vi "Filtered_read_of_file.vi"(4 "Data string":string, 5 "End Of File already Reached?":bool, 6 "Start of data (bytes)":i32, 7 "Desired Channel names":string[](array[string]), 8 "Valid Channel Options":string[][](array[string]), 9 "All Channels Present":string[](array[string]), 10 "Filename":path) -> (2 "Output Values":string[][](array[string]))   [LabVIEW 2010]
uses:
  Data_plotting_vis/Results_plotter_Global.vi
panel:
  out "Case":string
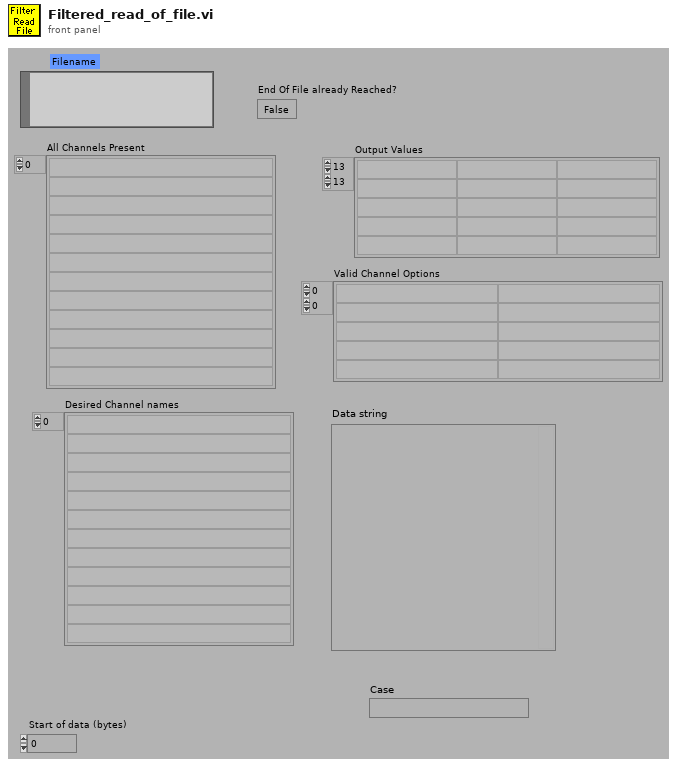
[diagram p1: front panel]
types:
  T1 = enum16{"read/write", "read-only", "write-only", "write-only (truncate)"}
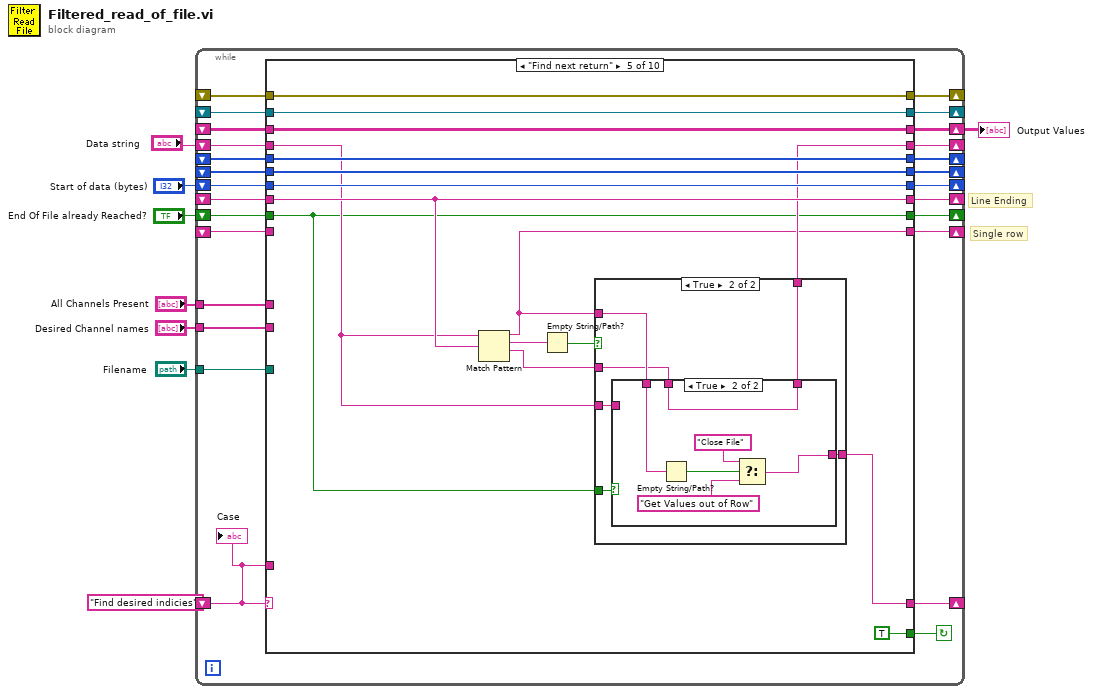
[diagram p0: block diagram]
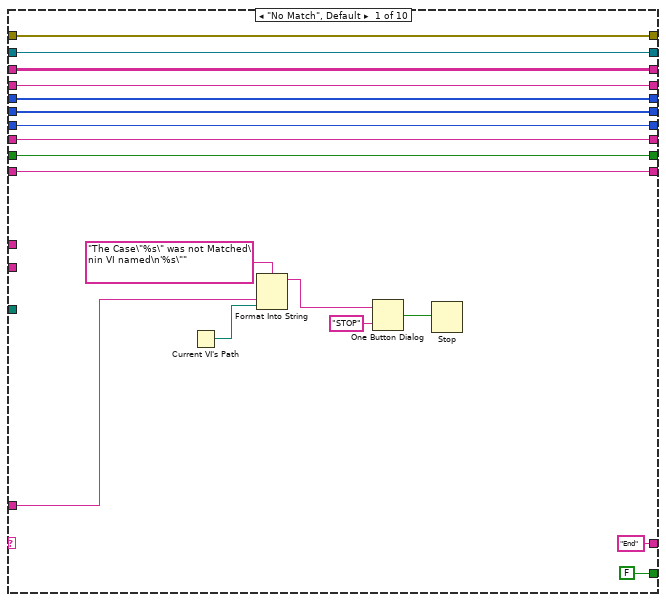
[diagram p2: hidden frame]
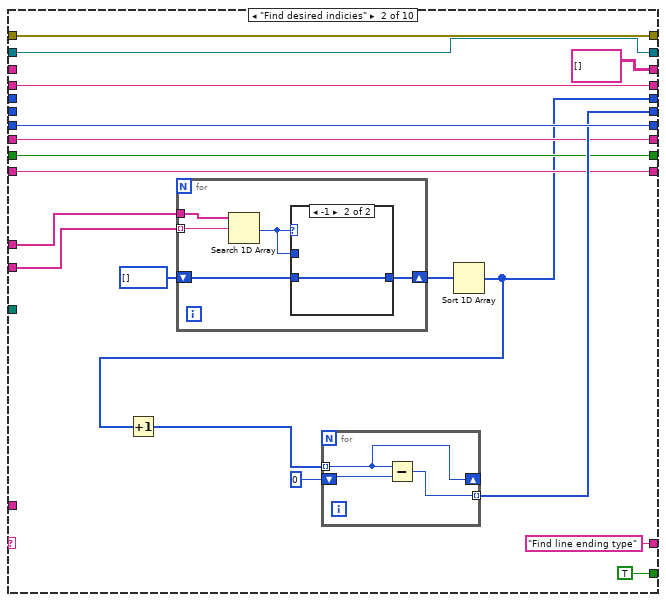
[diagram p3: hidden frame]
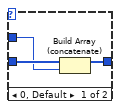
[diagram p4: hidden frame]
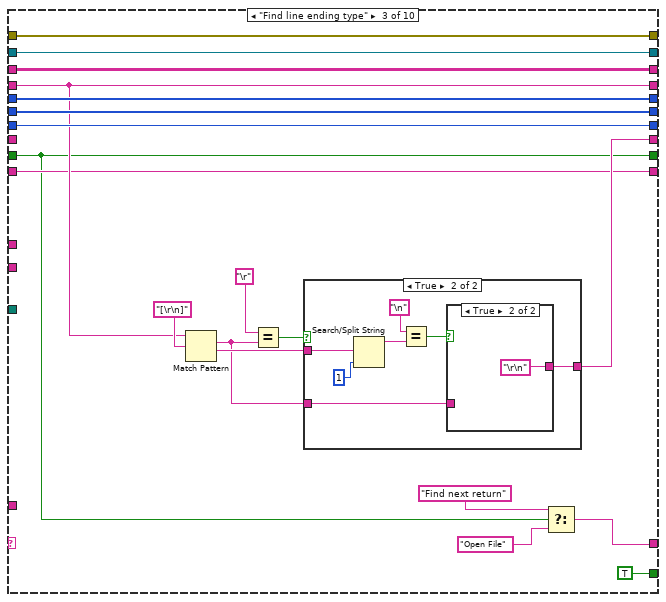
[diagram p5: hidden frame]
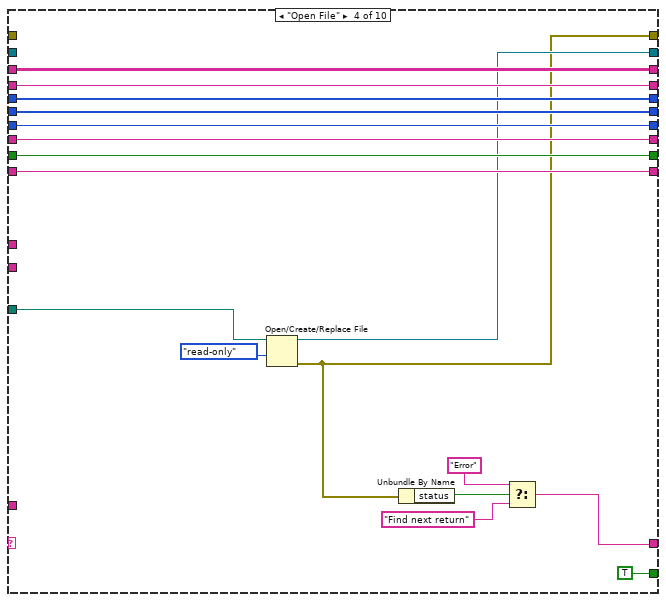
[diagram p8: hidden frame]
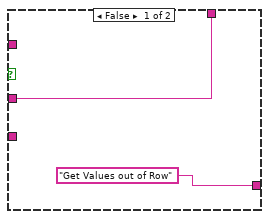
[diagram p9: hidden frame]
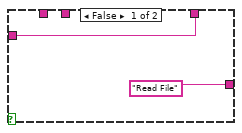
[diagram p10: hidden frame]
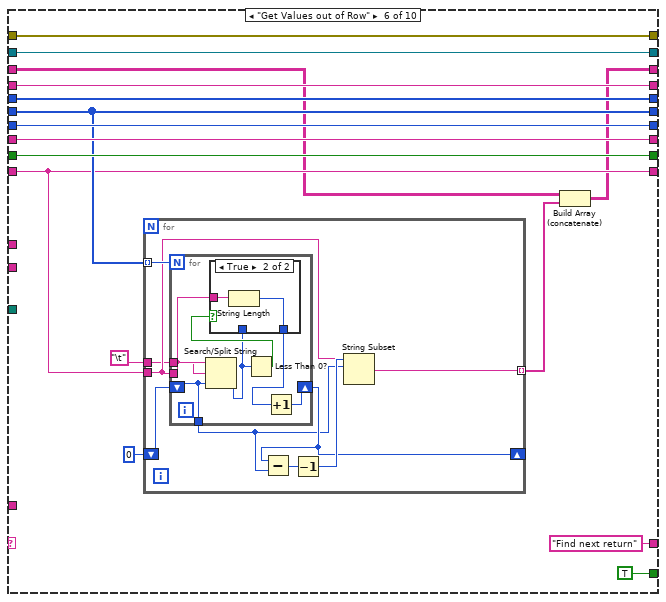
[diagram p11: hidden frame]
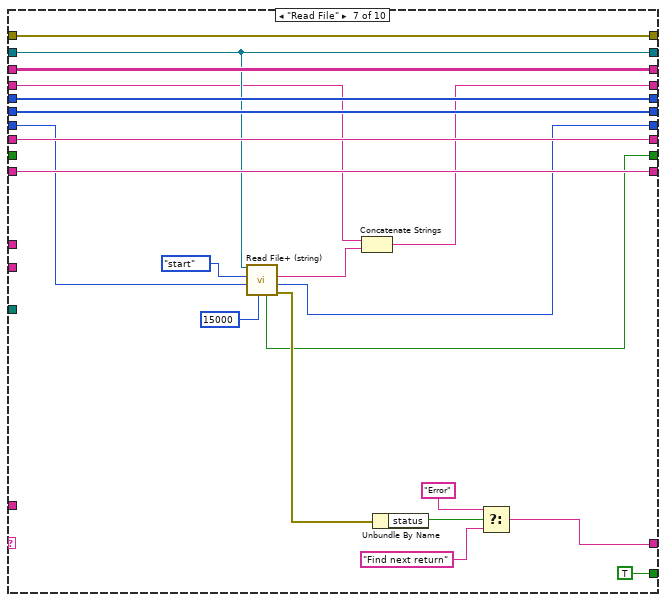
[diagram p13: hidden frame]
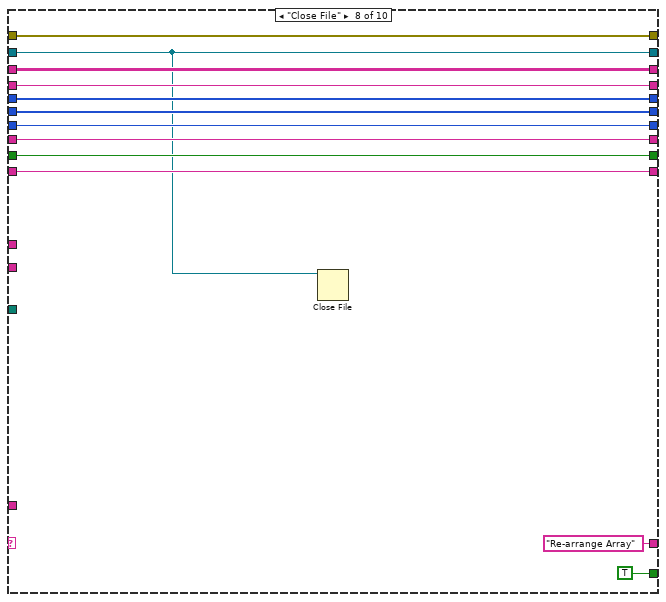
[diagram p14: hidden frame]
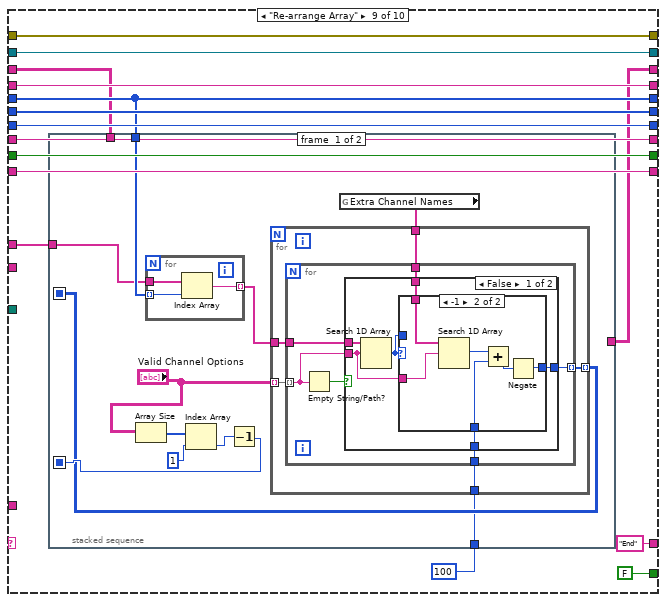
[diagram p15: hidden frame]
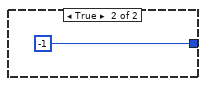
[diagram p17: hidden frame]
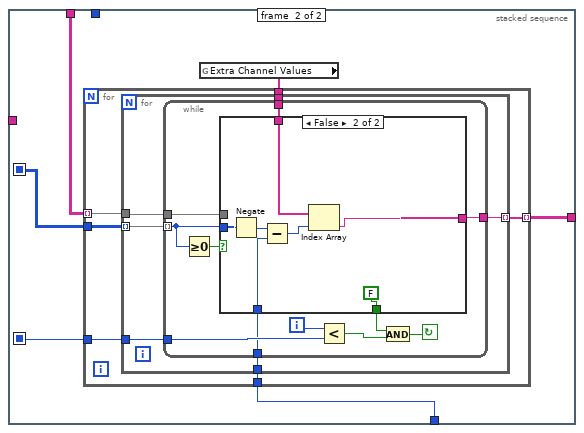
[diagram p18: hidden frame]
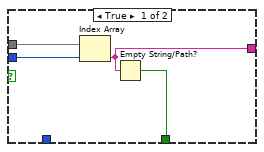
[diagram p19: hidden frame]
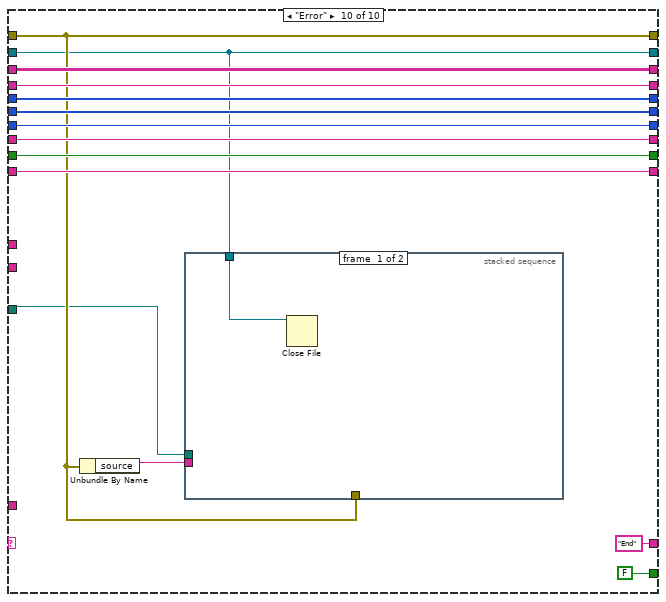
[diagram p20: hidden frame]
diagram:
  # "Single row"
  # "Line Ending"
  n1 = while {
    tunnel: "Filename" -> [w10]
    shift-left: _ -> [w12]
    shift-right: [w11] -> _
    shift-left: _ -> [w14]
    shift-right: [w13] -> _
    shift-left: _ -> [w16]
    shift-right: [w15] -> w2
    shift-left: "End Of File already Reached?" -> [w18]
    shift-right: [w17] -> _
    shift-left: _ -> [w19]
    shift-right: [w20] -> _
    shift-left: _ -> [w21]
    shift-right: [w22] -> _
    tunnel: "All Channels Present" -> [w23]
    tunnel: "Desired Channel names" -> [w9]
    shift-left: "Data string" -> [w25]
    shift-right: [w24] -> _
    shift-left: _ -> [w27]
    shift-right: [w26] -> _
    shift-left: "Start of data (bytes)" -> [w29]
    shift-right: [w28] -> _
    shift-left: _ -> [w30]
    shift-right: [w31] -> _
    shift-left: "Find desired indicies" -> [w33]
    shift-right: [w32] -> _
    stop <- w34 continue-if-true
    n2 = case shown="\"Find next return\"" w33 {
      tunnel: [FALSE ("Results File?") TRUE ("Results File?") TRUE ("Results File?") TRUE ("Results File?") TRUE ("Results File?") TRUE ("Results File?") TRUE ("Results File?") TRUE ("Results File?") FALSE ("Results File?") FALSE ("Results File?")] -> w34
      tunnel: w33 -> [w47 _ _ _ _ _ _ _ _ _]
      tunnel: ["End" "Find line ending type" ("f") w83 w113 w132 "Find next return" ("f") w200 "Re-arrange Array" ("f") "End" ("f") "End" ("f")] -> w32
      tunnel: [w44 w61 w100 w126 w143 w169 w215 w226 w242 w334] -> w31
      tunnel: w30 -> [w44 _ w100 w126 w143 w169 w215 w226 w242 w334]
      tunnel: w29 -> [w43 w68 w99 w125 w142 w174 w206 w225 w241 w333]
      tunnel: [w43 w68 w99 w125 w142 w174 w205 w225 w241 w333] -> w28
      tunnel: w27 -> [w42 _ w101 w127 w144 w175 w216 w227 w233 w335]
      tunnel: [w42 w54 w101 w127 w144 w175 w216 w227 w233 w335] -> w26
      tunnel: w25 -> [w41 w67 w93 w128 w136 w176 w198 w228 w243 w336]
      tunnel: [w41 w67 w93 w128 w137 w176 w196 w228 w243 w336] -> w24
      tunnel: w9 -> [_ w64 _ _ _ _ _ _ _ _]
      tunnel: w23 -> [_ w63 _ _ _ _ _ _ w232 _]
      tunnel: [w40 w60 w91 w123 w140 w171 w213 w223 w239 w330] -> w22
      tunnel: w21 -> [w40 w60 _ w123 w140 w171 w213 w223 w239 w330]
      tunnel: [w39 w59 w90 w122 w129 w168 w212 w222 w238 w329] -> w20
      tunnel: w19 -> [w39 w59 w90 w122 _ w168 w212 w222 w238 w329]
      tunnel: w18 -> [w38 w58 w84 w121 w131 w170 _ w221 w237 w328]
      tunnel: [w38 w58 w84 w121 w131 w170 w199 w221 w237 w328] -> w17
      tunnel: w16 -> [w37 _ w89 w120 w135 w164 w211 w220 w231 w327]
      tunnel: [w37 string[][] [] w89 w120 w135 w163 w211 w220 w230 w327] -> w15
      tunnel: w14 -> [w36 w56 w88 _ w134 w162 w207 w218 w235 w323]
      tunnel: [w36 w56 w88 w118 w134 w162 w207 w218 w235 w323] -> w13
      tunnel: w12 -> [w35 w55 w87 _ w133 w161 w208 w219 w236 w326]
      tunnel: [w35 w55 w87 w117 w133 w161 w208 w219 w236 w326] -> w11
      tunnel: w10 -> [_ _ _ w112 _ _ _ _ _ w324]
      frame "No Match", Default {
        n3 = Current VI's Path() -> (path=w48:path)
        n4 = Format Into String(format string="The Case\"%s\" was not Matched\nin VI named\n'%s\"" ("Format String"), w47, w48) -> (resulting string=w51:string)  [unwired: 2 in, 1 out]
        n5 = One Button Dialog(message=w51, button name ("OK")="STOP") -> (true=w49:bool)
        n6 = Stop(stop? (T)=w49) -> ()
      }
      frame "Find desired indicies" {
        n7 = for {
          tunnel: w63 -> [w78]
          tunnel: w64 -> [w77] mode=indexing
          shift-right: [w75] -> w66
          shift-left: i32[] [] -> [w76]
          n8 = Search 1D Array(1D array=w78, element=w77) -> (index of element=w74:i32)  [unwired: 1 in]
          n9 = case shown="-1" w74 {
            tunnel: w76 -> [w81 w82]
            tunnel: [w79 w82] -> w75
            tunnel: w74 -> [w80 _]
            frame 0, Default {
              n10 = Build Array (concatenate)(w81, w80) -> (w79:i32[])
            }
            frame -1 {
            }
          }
        }
        n11 = Sort 1D Array(array=w66) -> (sorted array=w54:i32[])
        n12 = Increment(x=w54) -> (x+1=w53:i32[])
        n13 = for {
          shift-right: [w72] -> _
          shift-left: 0 -> [w73]
          tunnel: w53 -> [w72] mode=indexing
          tunnel: [w71] -> w61 mode=indexing
          n14 = Subtract(x=w72, y=w73) -> (x-y=w71:i32)
        }
      }
      frame "Find line ending type" {
        n15 = Match Pattern(string=w93, regular expression="[\r\n]") -> (match substring=w92:string, after substring=w97:string)  [unwired: 1 in, 2 out]
        n16 = Equal?(x="\r" ("regular expression"), y=w92) -> (x = y?=w96:bool)
        n17 = case shown="True" w96 {
          tunnel: w97 -> [_ w106]
          tunnel: w92 -> [w102 w103]
          tunnel: [w102 w104] -> w91
          frame False {
          }
          frame True {
            n18 = Search/Split String(string=w106, offset (0)=1) -> (substring before match=w107:string)  [unwired: 1 in, 2 out]
            n19 = Equal?(x="\n" ("regular expression"), y=w107) -> (x = y?=w105:bool)
            n20 = case shown="True" w105 {
              tunnel: [w110 "\r\n" ("regular expression")] -> w104
              tunnel: w103 -> [w110 _]
              frame False {
              }
              frame True {
              }
            }
          }
        }
        n21 = Select(t="Find next return", s=w84, f="Open File") -> (s? t:f=w83:string)
      }
      frame "Open File" {
        n22 = Open/Create/Replace File(file path (use dialog)=w112, access (0:read/write)=T1."read-only" ("open mode (0)")) -> (refnum out=w118:refnum<file>, error out=w117:errorcluster)  [unwired: 4 in, 1 out]
        n23 = Unbundle By Name(w117) -> ("status"=w114:bool)
        n24 = Select(t="Error", s=w114, f="Find next return") -> (s? t:f=w113:string)
      }
      frame "Find next return" {
        n25 = Match Pattern(string=w136, regular expression=w140) -> (before substring=w129:string, match substring=w139:string, after substring=w130:string)  [unwired: 1 in, 1 out]
        n26 = Empty String/Path?(string/path=w139) -> (empty?=w138:bool)
        n27 = case shown="True" w138 {
          tunnel: [w146 w150] -> w137
          tunnel: w130 -> [w146 w147]
          tunnel: w136 -> [_ w149]
          tunnel: ["Get Values out of Row" ("f") w151] -> w132
          tunnel: w131 -> [_ w152]
          tunnel: w129 -> [_ w148]
          frame False {
          }
          frame True {
            n28 = case shown="True" w152 {
              tunnel: ["Read File" ("f") w157] -> w151
              tunnel: w148 -> [_ w156]
              tunnel: [w153 w155] -> w150
              tunnel: w149 -> [w153 _]
              tunnel: w147 -> [_ w155]
              frame False {
              }
              frame True {
                n29 = Empty String/Path?(string/path=w156) -> (empty?=w160:bool)
                n30 = Select(t="Close File", s=w160, f="Get Values out of Row") -> (s? t:f=w157:string)
              }
            }
          }
        }
      }
      frame "Get Values out of Row" {
        n31 = for {
          tunnel: w169 -> [w185] mode=indexing
          shift-right: [w180] -> _
          shift-left: 0 -> [w184]
          tunnel: w168 -> [w181]
          tunnel: "\t" -> [w178]
          tunnel: [w177] -> w165 mode=indexing
          n32 = for {
            N: w185 -> [_]
            shift-right: [w191] -> w180
            shift-left: w184 -> [w192]
            tunnel: w181 -> [w189]
            tunnel: [w192] -> w179
            tunnel: w178 -> [w186]
            n33 = Search/Split String(string=w189, search string/char (-)=w186, offset (0)=w192) -> (offset of match=w187:i32)  [unwired: 2 out]
            n34 = Less Than 0?(x=w187) -> (x < 0?=w190:bool)
            n35 = case shown="True" w190 {
              tunnel: w189 -> [_ w195]
              tunnel: [w193 w194] -> w188
              tunnel: w187 -> [w193 _]
              frame False {
              }
              frame True {
                n36 = String Length(string=w195) -> (length=w194:i32)
              }
            }
            n37 = Increment(x=w188) -> (x+1=w191:i32)
          }
          n38 = Subtract(x=w180, y=w179) -> (x-y=w183:i32)
          n39 = Decrement(x=w183) -> (x-1=w182:i32)
          n40 = String Subset(string=w181, offset (0)=w179, length (rest)=w182) -> (substring=w177:string)
        }
        n41 = Build Array (concatenate)(w164, w165) -> (w163:string[][])
      }
      frame "Read File" {
        n42 = call <vilib>:"Read File+ (string).vi"("count"=15000, "pos offset (bytes:0)"=w206, "pos mode (rel. to current:2)"=enum16{"start", "end", "current"}."start", "refnum"=w207) -> ("error out"=w201:errorcluster, "mark after read (bytes)"=w205:i32, "string"=w197:string, "EOF?"=w199:bool)  [unwired: 3 in, 1 out]
        n43 = Concatenate Strings(w198, w197) -> (w196:string)
        n44 = Unbundle By Name(w201) -> ("status"=w202:bool)
        n45 = Select(t="Error", s=w202, f="Find next return") -> (s? t:f=w200:string)
      }
      frame "Close File" {
        n46 = Close File(refnum=w218) -> ()  [unwired: 1 in, 2 out]
      }
      frame "Re-arrange Array" {
        n47 = stacked-sequence {
          seq-local: [w247 _] -> [_ w286]
          seq-local: [w246 _] -> [_ w287]
          tunnel: w233 -> [w253 _]
          tunnel: w232 -> [w252 _]
          tunnel: w231 -> [_ w288]
          tunnel: [_ w285] -> w230
          tunnel: 100 ("y") -> [w245 w284]
          frame #0 {
            n48 = Array Size(array="Valid Channel Options") -> (size(s)=w250:i32[])
            n49 = for {
              tunnel: w253 -> [w282] mode=indexing
              tunnel: w252 -> [w281]
              tunnel: [w280] -> w254 mode=indexing
              n50 = Index Array(array=w281, index=w282) -> (element=w280:string)
            }
            n51 = Index Array(array=w250, index=1 ("Index")) -> (element=w248:i32)
            n52 = Decrement(x=w248) -> (x-1=w247:i32)
            n53 = global read "Results_plotter_Global.vi" "Extra Channel Names"() -> (w244:string[])
            n54 = for {
              tunnel: w254 -> [w259]
              tunnel: "Valid Channel Options" -> [w258] mode=indexing
              tunnel: [w257] -> w246 mode=indexing
              tunnel: w245 -> [w256]
              tunnel: w244 -> [w255]
              n55 = for {
                tunnel: w258 -> [w263] mode=indexing
                tunnel: w259 -> [w265]
                tunnel: [w264] -> w257 mode=indexing
                tunnel: w256 -> [w261]
                tunnel: w255 -> [w260]
                n56 = Empty String/Path?(string/path=w263) -> (empty?=w262:bool)
                n57 = case shown="False" w262 {
                  tunnel: w265 -> [w271 _]
                  tunnel: [w269 -1 ("index of element")] -> w264
                  tunnel: w263 -> [w270 _]
                  tunnel: w261 -> [w267 _]
                  tunnel: w260 -> [w266 _]
                  frame False {
                    n58 = Search 1D Array(1D array=w271, element=w270) -> (index of element=w268:i32)  [unwired: 1 in]
                    n59 = case shown="-1" w268 {
                      tunnel: w270 -> [_ w278]
                      tunnel: [w272 w275] -> w269
                      tunnel: w268 -> [w272 _]
                      tunnel: w267 -> [_ w274]
                      tunnel: w266 -> [_ w273]
                      frame 0, Default {
                      }
                      frame -1 {
                        n60 = Search 1D Array(1D array=w273, element=w278) -> (index of element=w277:i32)  [unwired: 1 in]
                        n61 = Add(x=w277, y=w274) -> (x+y=w276:i32)
                        n62 = Negate(x=w276) -> (-x=w275:i32)
                      }
                    }
                  }
                  frame True {
                  }
                }
              }
            }
          }
          frame #1 {
            n63 = global read "Results_plotter_Global.vi" "Extra Channel Values"() -> (w283:string[])
            n64 = for {
              tunnel: w287 -> [w294]
              tunnel: w288 -> [w293] mode=indexing
              tunnel: [w292] -> w285 mode=indexing
              tunnel: w286 -> [w291]
              tunnel: w284 -> [w290]
              tunnel: w283 -> [w289]
              n65 = for {
                tunnel: w294 -> [w298] mode=indexing
                tunnel: w293 -> [w300]
                tunnel: [w299] -> w292 mode=indexing
                tunnel: w291 -> [w297]
                tunnel: w290 -> [w296]
                tunnel: w289 -> [w295]
                n66 = while {
                  tunnel: w295 -> [w301]
                  tunnel: w296 -> [w302]
                  tunnel: w297 -> [w308]
                  tunnel: w298 -> [w304] mode=indexing
                  tunnel: [w310] -> w299
                  tunnel: w300 -> [w311]
                  i -> [w309]
                  stop <- w306 continue-if-true
                  n67 = Greater Or Equal To 0?(x=w304) -> (x >= 0?=w303:bool)
                  n68 = case shown="False" w303 {
                    tunnel: w311 -> [w315 _]
                    tunnel: [w313 w322] -> w310
                    tunnel: w304 -> [w314 w321]
                    tunnel: [w312 FALSE] -> w305
                    tunnel: w302 -> [_ w319]
                    tunnel: w301 -> [_ w316]
                    frame True {
                      n69 = Index Array(array=w315, index=w314) -> (element=w313:string)
                      n70 = Empty String/Path?(string/path=w313) -> (empty?=w312:bool)
                    }
                    frame False {
                      n71 = Negate(x=w321) -> (-x=w320:i32)
                      n72 = Subtract(x=w320, y=w319) -> (x-y=w318:i32)
                      n73 = Index Array(array=w316, index=w318) -> (element=w322:string)
                    }
                  }
                  n74 = Less?(x=w309, y=w308) -> (x < y?=w307:bool)
                  n75 = And(x=w305, y=w307) -> (x .and. y?=w306:bool)
                }
              }
            }
          }
        }
      }
      frame "Error" {
        n76 = Unbundle By Name(w326) -> ("source"=w325:string)
        n77 = stacked-sequence {
          tunnel: w326 -> [_ w343]
          tunnel: w325 -> [_ w342]
          tunnel: w324 -> [_ w341]
          tunnel: w323 -> [w337 _]
          frame #0 {
            n78 = Close File(refnum=w337) -> ()  [unwired: 1 in, 2 out]
          }
          frame #1 {
            w344 = FALSE  # Dialog Box (T)
            n79 = Format Into String(format string="Whilst reading from filename \"%s\"\n%s" ("Format String"), w341, w342) -> (resulting string=w339:string)  [unwired: 2 in, 1 out]
            n80 = Bundle By Name(cluster=w343, "source"=w339) -> (w338:errorcluster)
            n81 = call "EnFlo_Error_Handler.vi"("error in (no error)"=w338, "Error Type"="File Error", "Dialog Box (T)"=w344) -> ()  [unwired: 3 out]
          }
        }
      }
    }
    "Case" <- w33
  }
  "Output Values" <- w2
